vi "get channels from line.vi"() -> ()   [LabVIEW 2015, in "TDMS datalogger configuration.lvclass"]
uses:
  TDMS datalogger configuration.lvclass
  <vilib>/NI/Tag Bus Module Framework/channel/TBM channel.lvclass
panel:
  in  "Line":T1
  out "Channels":refnum<class "TBM channel.lvclass">[](array[class])
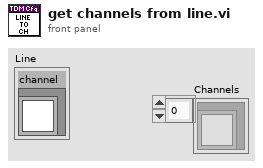
[diagram p1: front panel]
types:
  T1 = cluster{"channel":refnum<class "TBM channel.lvclass">}
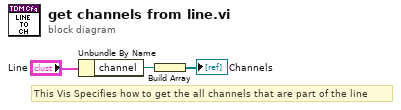
[diagram p0: block diagram]
diagram:
  # "This Vis Specifies how to get the all channels that are part of the line"
  n1 = Unbundle By Name("Line") -> ("channel"=w2:refnum<class "TBM channel.lvclass">)
  n2 = Build Array(w2) -> (→"Channels":refnum<class "TBM channel.lvclass">[])
